vi "Get Waveform dt Values.vi"(8 "error in (no error)":errorcluster, 10 "waveform paths":string[](array[string]), 11 "WaveformStreaming in":T1) -> (0 "error out":errorcluster, 2 "dt values":dbl[](array[numeric]), 3 "WaveformStreaming out":T1)   [LabVIEW 2020, in "NI_VS Waveform Streaming Interface.lvlib"]
doc: "Returns an array of the delta T values for the specified waveform(s)."
uses:
  <vilib>/NI VeriStand/Execution/WaveformStreaming/NI_VS Waveform Streaming Interface.lvlib
  <vilib>/NI VeriStand/Execution/WaveformStreaming/WaveformStreamingAPI.ctl
  NationalInstruments.VeriStand.ClientAPI
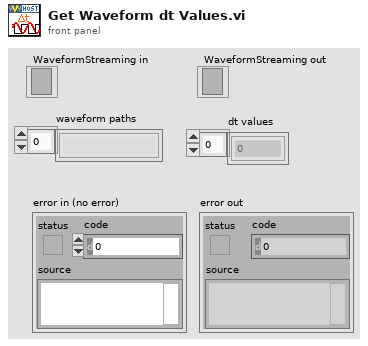
[diagram p1: front panel]
types:
  T1 = typedef "NI_VS Waveform Streaming Interface.lvlib/WaveformStreamingAPI.ctl" = refnum<k24>
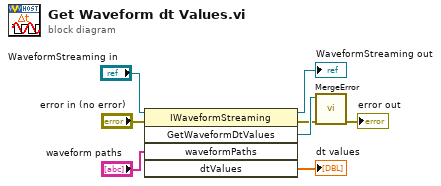
[diagram p0: block diagram]
diagram:
  n1 = invoke class="IWaveformStreaming" method="GetWaveformDtValues"(reference="WaveformStreaming in", error in="error in (no error)", "waveformPaths"="waveform paths") -> (reference out=→"WaveformStreaming out":T1, error out=w3:errorcluster, "GetWaveformDtValues"=w4:refnum<k24>, "dtValues"=→"dt values":dbl[])  [unwired: 2 in, 1 out]
  n2 = call <vilib>:"MergeError.vi"("error in (no error)"=w3, "Error"=w4) -> ("error out"=→"error out":errorcluster)  [unwired: 9 in]
